vi "AlazarCoprocessorRegisterWrite.vi"(3 "error in (no error)":errorcluster, 4 "Value":u32, 5 "Offset":u32, 6 "Handle":u64) -> (0 "error out":errorcluster, 1 "Return Code":u32, 2 "Handle":u64)   [LabVIEW 2009]
doc: "Write a value to a user-programmable coprocessor FPGA register."
uses:
  ATSApi.dll
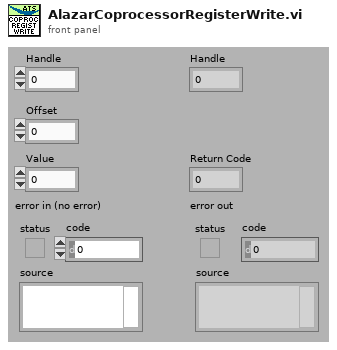
[diagram p1: front panel]
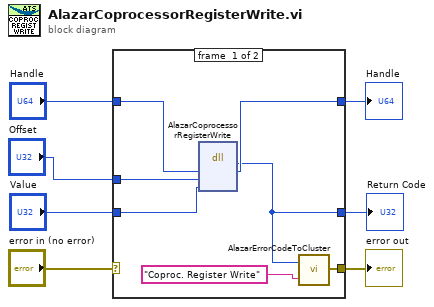
[diagram p0: block diagram]
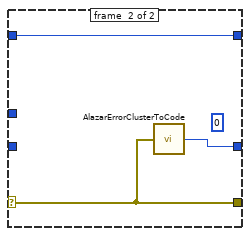
[diagram p2: hidden frame]
diagram:
  n1 = case shown="No Error" "error in (no error)" {
    selector: "error in (no error)" -> [_ w17]
    tunnel: [w10 w17] -> w6
    tunnel: [w9 w16] -> w5
    tunnel: "Handle" -> [w14 w15]
    tunnel: [w13 w15] -> w3
    tunnel: "Offset" -> [w12 _]
    tunnel: "Value" -> [w11 _]
    frame #0 {
      n2 = dll-call lib="ATSApi.dll" fn="AlazarCoprocessorRegisterWrite"("handle"=w14, "offset"=w12, "value"=w11) -> ("return type"=w9:u32, "handle"=w13:u64)  [unwired: 5 in, 2 out]
      n3 = call "AlazarErrorCodeToCluster.vi"("Message"="Coproc. Register Write", "Error Code"=w9) -> ("error out"=w10:errorcluster)
    }
    frame #1 {
      (unwired) u32 0
      n4 = call "AlazarErrorClusterToCode.vi"("error in (no error)"=w17) -> ("Error Code"=w16:u32)
    }
  }
  "Handle" <- w3
  "error out" <- w6
  "Return Code" <- w5
